vi "Get Formatting Settings - Backgrounds - Inline.vi"(8 "error in (no error)":errorcluster {"code" format="Error %.0f"}, 11 "VIDoc Printer In":refnum<class "VIDoc Printer.lvclass">) -> (0 "error out":errorcluster {"code" format="Error %.0f"}, 2 "Background Formatting":T1, 3 "VIDoc Printer Out":refnum<class "VIDoc Printer.lvclass">)   [LabVIEW 2023, in "VIDoc Printer.lvlib" / "VIDoc Printer.lvclass"]
uses:
  VIDoc Printer.lvclass
  Settings/Printer Settings/Background Formatting Cluster.ctl
  VIDoc Printer.lvclass/VIDoc Printer.ctl
  Settings/Printer Settings/Printer Settings.lvclass
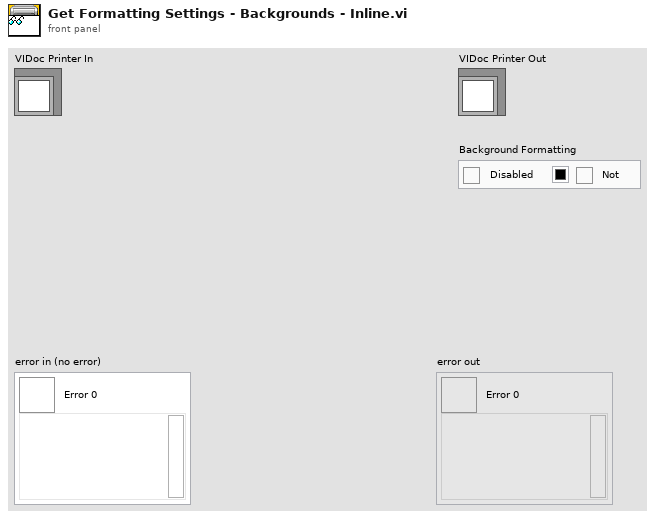
[diagram p1: front panel]
types:
  T1 = typedef "VIDoc Printer.lvlib/Printer Settings.lvclass/Background Formatting Cluster.ctl" = cluster{"Option":bool, "Color":u32, "Operator":bool}
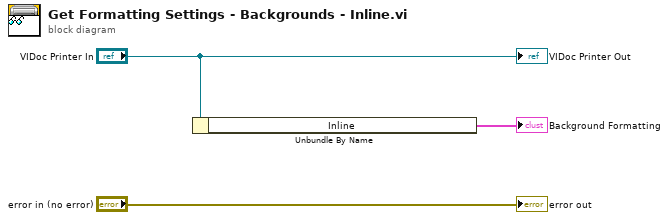
[diagram p0: block diagram]
diagram:
  n1 = Unbundle By Name("VIDoc Printer In") -> ("Inline"=→"Background Formatting":T1)
  "error out" <- "error in (no error)"
  "VIDoc Printer Out" <- "VIDoc Printer In"
